vi "CAlex2_SetCuff_Hip_TreadmillLeft.vi"(8 "Hip Cuff Forward Shift (m)":dbl, 9 "Hip Cuff Height (m)":dbl, 10 "Hip Cuff Width (m)":dbl, 11 "Hip Width (m)":dbl) -> (3 "Hip Cuff":T1={"BodyID"=0, "CoM(CuffCS)"={"Coord4"=[0.0, 0.0, 0.0, 1.0], "ID"=0}, "Mass(kg)"=0.0, "CablePts(CuffCS)"=[], "Cuff->Body"=[[1.0, 0.0, 0.0, 0.0], [0.0, 1.0, 0.0, 0.0], [0.0, 0.0, 1.0, 0.0], [0.0, 0.0, 0.0, 1.0]]})   [LabVIEW 2016, in "CAlex2.lvclass"]
uses:
  CAlex2.lvclass
  SerialChain-Cable/TypeDef/Cuff.ctl
  SerialChain/TypeDef/PointOnBody.ctl
  <vilib>/Analysis/Matrix/Datatypes/RealMatrix.ctl
  SerialChain/TypeDef/xyzO.ctl
  SerialChain/SerialChain.lvclass
  <vilib>/Analysis/Matrix/NI_Matrix.lvlib
  SerialChain-Cable/SerialChain-Cable.lvclass
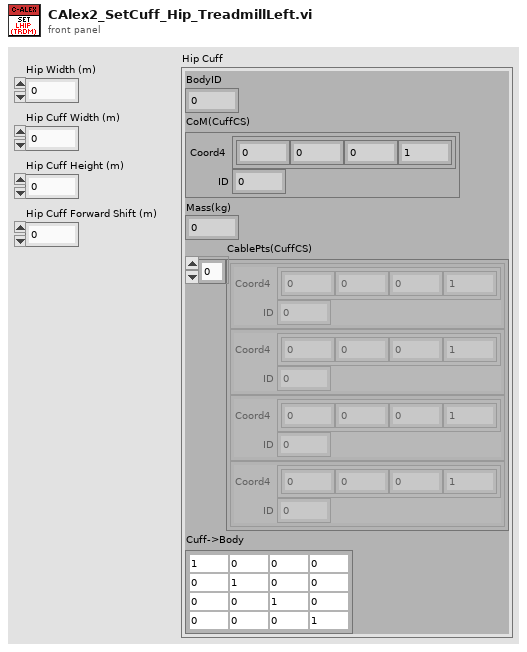
[diagram p1: front panel]
types:
  T1 = typedef "SerialChain-Cable.lvclass/Cuff.ctl" = cluster{"BodyID":i32, "CoM(CuffCS)":T2, "Mass(kg)":dbl, "CablePts(CuffCS)":T2[], "Cuff->Body":T3}
  T2 = typedef "SerialChain.lvclass/PointOnBody.ctl" = cluster{"Coord4":dbl[], "ID":i32}
  T3 = typedef "NI_Matrix.lvlib/RealMatrix.ctl" = dbl[][]
  T4 = typedef "SerialChain.lvclass/xyzO.ctl" = enum16{"X", "Y", "Z", "O"}
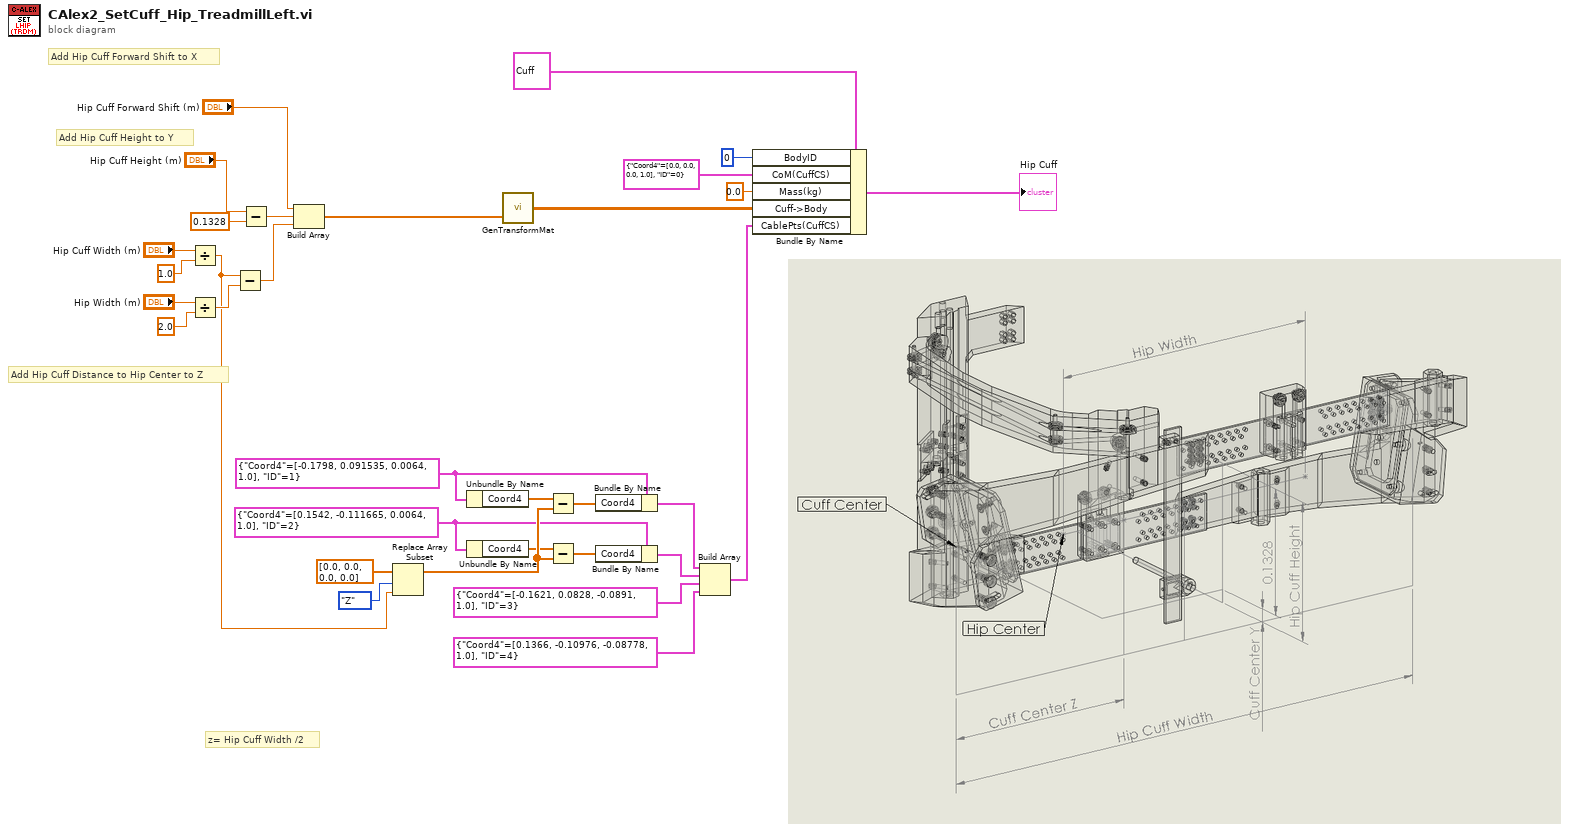
[diagram p0: block diagram]
diagram:
  w7 = T2 {"Coord4"=[-0.1798, 0.091535, 0.0064, 1.0], "ID"=1} ("CoM(CuffCS)")
  w6 = T2 {"Coord4"=[0.1542, -0.111665, 0.0064, 1.0], "ID"=2} ("CoM(CuffCS)")
  # "Add Hip Cuff Distance to Hip Center to Z"
  # "Add Hip Cuff Forward Shift to X"
  # "z= Hip Cuff Width /2"
  # "Add Hip Cuff Height to Y"
  n1 = Divide(x="Hip Cuff Width (m)", y=1.0) -> (x/y=w11:dbl)
  n2 = Divide(x="Hip Width (m)", y=2.0) -> (x/y=w12:dbl)
  n3 = Subtract(x=w11, y=w12) -> (x-y=w10:dbl)
  n4 = Subtract(x="Hip Cuff Height (m)", y=0.1328) -> (x-y=w2:dbl)
  n5 = Build Array("Hip Cuff Forward Shift (m)", w2, w10) -> (w5:dbl[])
  n6 = Replace Array Subset(array=dbl[] [0.0, 0.0, 0.0, 0.0] ("Coord4"), new element=w11, index=xyzO."Z" ("XYZ")) -> (w26:dbl[])
  n7 = Unbundle By Name(w7) -> ("Coord4"=w22:dbl[])
  n8 = Unbundle By Name(w6) -> ("Coord4"=w25:dbl[])
  n9 = call "GenTransformMat.vi"("Translate 3Vector"=w5) -> ("Transformation Matrix"=w4:T3)  [unwired: 1 in]
  n10 = Subtract(x=w22, y=w26) -> (x-y=w27:dbl[])
  n11 = Subtract(x=w25, y=w26) -> (x-y=w28:dbl[])
  n12 = Bundle By Name(cluster=w7, "Coord4"=w27) -> (w18:T2)
  n13 = Bundle By Name(cluster=w6, "Coord4"=w28) -> (w19:T2)
  n14 = Build Array(w18, w19, T2 {"Coord4"=[-0.1621, 0.0828, -0.0891, 1.0], "ID"=3} ("CoM(CuffCS)"), T2 {"Coord4"=[0.1366, -0.10976, -0.08778, 1.0], "ID"=4} ("CoM(CuffCS)")) -> (w17:T2[])
  n15 = Bundle By Name(cluster=T1 {"BodyID"=0, "CoM(CuffCS)"={"Coord4"=[0.0, 0.0, 0.0, 1.0], "ID"=0}, "Mass(kg)"=0.0, "CablePts(CuffCS)"=[], "Cuff->Body"=[[1.0, 0.0, 0.0, 0.0], [0.0, 1.0, 0.0, 0.0], [0.0, 0.0, 1.0, 0.0], [0.0, 0.0, 0.0, 1.0]]} ("Cuff Design"), "BodyID"=0, "CoM(CuffCS)"=T2 {"Coord4"=[0.0, 0.0, 0.0, 1.0], "ID"=0}, "Mass(kg)"=0.0, "Cuff->Body"=w4, "CablePts(CuffCS)"=w17) -> (→"Hip Cuff":T1)
